vi "Create AIs.vi"(0 "reference in":refnum<class "Stand.lvclass">, 11 "error in (no error)":errorcluster) -> (4 "reference out":refnum<class "Stand.lvclass">, 15 "error out":errorcluster)   [LabVIEW 2019, in "Stand.lvclass"]
uses:
  Stand.lvclass
  C:/Users/ANENKOV_V1/Desktop/src/Proccess_class/Proccess.lvclass
  C:/Users/ANENKOV_V1/Desktop/src/Device_class/Device.lvclass
  Stand.lvclass/Stand.ctl
  TypeDef/CalibrationData.ctl
  TypeDef/GUI Setting Channel.ctl
  TypeDef/GUI AI Ranges.ctl
  TypeDef/Scale Data.ctl
  Device_class/Device.lvclass/Device.ctl
  Proccess_class/Proccess.lvclass/Proccess.ctl
  SV_Puplisher_class/SV_Publisher.lvclass/SV_Publisher.ctl
  AI_class/AI.lvclass
  Proccess_class/TAGs.ctl
  PiecedLinearScale_class/Scale_PiecedLinear.lvclass
  TypeDef/ConfigAnalogComp.ctl
  AI_class/AI Alarm Type.ctl
  PiecedLinearScale_class/Scale_PiecedLinear.lvclass/Scale_PiecedLinear.ctl
  AI_class/AI.lvclass/AI.ctl
  AnalogComparator_class/AnalogComparator.lvclass/AnalogComparator.ctl
  0edcd56b-ce9e-46cf-b3ab-c0e0e087750b.vi
  <vilib>/Utility/error.llb/Clear Errors.vi
  SV_Puplisher_class/Set SV.vi/1ae5d02c-efd0-450a-8aa4-8388e25d05bc.vi
  AnalogComparator_class/SetConfig.vi
  ConfigInterface_class/ConfigInterface.lvclass
  Proccess_class/Proccess.lvclass
  Device_class/Device.lvclass
  SV_Puplisher_class/SV_Publisher.lvclass
  AnalogComparator_class/AnalogComparator.lvclass
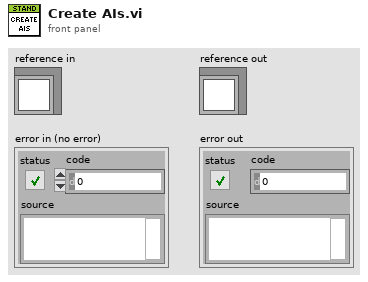
[diagram p1: front panel]
types:
  T1 = typedef "CalibrationData.ctl" = cluster{"Channels":T2[], "Scales":T4[]}
  T2 = typedef "GUI Setting Channel.ctl" = cluster{"Name":string, "AI Ranges":T3, "ScaleIndex":u32}
  T3 = typedef "GUI AI Ranges.ctl" = cluster{"HI":bool, "HIHI":bool, "LO":bool, "LOLO":bool, "HIHI VAL":dbl, "HI VAL":dbl, "LO VAL":dbl, "LOLO VAL":dbl, "MAX RAW":dbl, "MIN RAW":dbl, "MAX SCALED":dbl, "MIN SCALED":dbl}
  T4 = typedef "Scale Data.ctl" = cluster{"index":i32, "Name":string, "X":dbl[], "Y":dbl[]}
  T5 = typedef "Proccess.lvclass/TAGs.ctl" = cluster{"TAG":string, "PTAG":string, "DESC":string}
  T6 = typedef "ConfigAnalogComp.ctl" = cluster{"Threshold":dbl, "Hysteresis":dbl, "Invert":bool, "Enable":bool, "LockEn":bool}
  T7 = typedef "AnalogComparator.lvclass/AI Alarm Type.ctl" = enum16{"RAW MAX", "RAW MIN", "HIHI", "HI", "LO", "LOLO"}
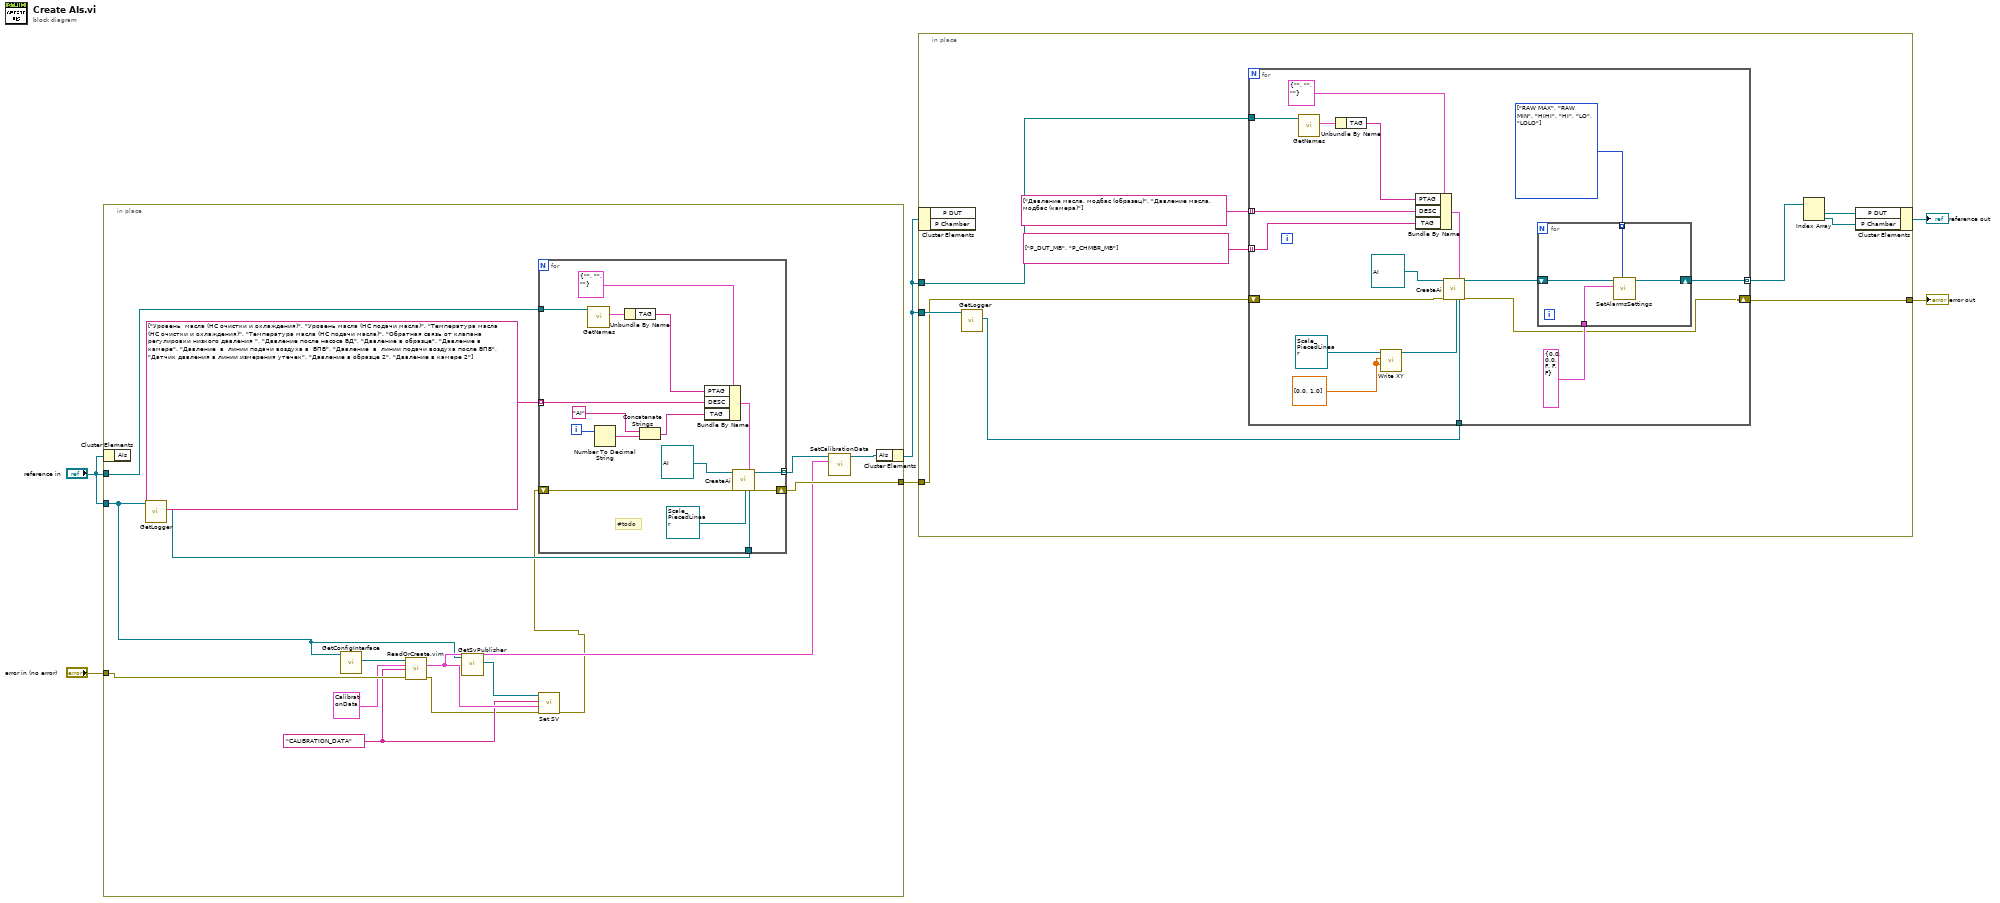
[diagram p0: block diagram]
diagram:
  n1 = in-place {
    in-place-border: "error in (no error)" -> [w15]
    in-place-border: "reference in" -> [w20]
    in-place-border: "reference in" -> [w16]
    in-place-border: [w18] -> w4
    w9 = "CALIBRATION_DATA" ("Name")
    n2 = in-place-cluster #1("reference in") -> ()  [unwired: 1 out]
    n3 = call "GetLogger.vi"("Proccess in"=w16) -> ("Logger"=w19:refnum<class "Logger.lvclass">)  [unwired: 10 in]
    n4 = call "GetConfigInterface.vi"("Device in"=w16) -> ("ConfigInterface"=w11:refnum<class "ConfigInterface.lvclass">)  [unwired: 10 in]
    n5 = call "ReadOrCreate.vim"("reference in"=w11, "Type and Defaults"=T1 {"Channels"=[{"Name"="AI0", "AI Ranges"={"HI"=FALSE, "HIHI"=FALSE, "LO"=FALSE, "LOLO"=FALSE, "HIHI VAL"=0.0, "HI VAL"=90.0, "LO VAL"=10.0, "LOLO VAL"=0.0, "MAX RAW"=20.0, "MIN RAW"=4.0, "MAX SCALED"=20.0, "MIN SCALED"=4.0}, "ScaleIndex"=0}, {"Name"="AI1", "AI Ranges"={"HI"=FALSE, "HIHI"=FALSE, "LO"=FALSE, "LOLO"=FALSE, "HIHI VAL"=0.0, "HI VAL"=90.0, "LO VAL"=10.0, "LOLO VAL"=0.0, "MAX RAW"=20.0, "MIN RAW"=4.0, "MAX SCALED"=20.0, "MIN SCALED"=4.0}, "ScaleIndex"=0}, {"Name"="AI2", "AI Ranges"={"HI"=FALSE, "HIHI"=FALSE, "LO"=FALSE, "LOLO"=FALSE, "HIHI VAL"=0.0, "HI VAL"=90.0, "LO VAL"=10.0, "LOLO VAL"=0.0, "MAX RAW"=20.0, "MIN RAW"=4.0, "MAX SCALED"=20.0, "MIN SCALED"=4.0}, "ScaleIndex"=0}, {"Name"="AI3", "AI Ranges"={"HI"=FALSE, "HIHI"=FALSE, "LO"=FALSE, "LOLO"=FALSE, "HIHI VAL"=0.0, "HI VAL"=90.0, "LO VAL"=10.0, "LOLO VAL"=0.0, "MAX RAW"=20.0, "MIN RAW"=4.0, "MAX SCALED"=20.0, "MIN SCALED"=4.0}, "ScaleIndex"=0}, {"Name"="AI4", "AI Ranges"={"HI"=FALSE, "HIHI"=FALSE, "LO"=FALSE, "LOLO"=FALSE, "HIHI VAL"=0.0, "HI VAL"=90.0, "LO VAL"=10.0, "LOLO VAL"=0.0, "MAX RAW"=20.0, "MIN RAW"=4.0, "MAX SCALED"=20.0, "MIN SCALED"=4.0}, "ScaleIndex"=0}, {"Name"="AI5", "AI Ranges"={"HI"=FALSE, "HIHI"=FALSE, "LO"=FALSE, "LOLO"=FALSE, "HIHI VAL"=0.0, "HI VAL"=90.0, "LO VAL"=10.0, "LOLO VAL"=0.0, "MAX RAW"=20.0, "MIN RAW"=4.0, "MAX SCALED"=20.0, "MIN SCALED"=4.0}, "ScaleIndex"=0}, {"Name"="AI6", "AI Ranges"={"HI"=FALSE, "HIHI"=FALSE, "LO"=FALSE, "LOLO"=FALSE, "HIHI VAL"=0.0, "HI VAL"=90.0, "LO VAL"=10.0, "LOLO VAL"=0.0, "MAX RAW"=20.0, "MIN RAW"=4.0, "MAX SCALED"=20.0, "MIN SCALED"=4.0}, "ScaleIndex"=0}, {"Name"="AI7", "AI Ranges"={"HI"=FALSE, "HIHI"=FALSE, "LO"=FALSE, "LOLO"=FALSE, "HIHI VAL"=0.0, "HI VAL"=90.0, "LO VAL"=10.0, "LOLO VAL"=0.0, "MAX RAW"=20.0, "MIN RAW"=4.0, "MAX SCALED"=20.0, "MIN SCALED"=4.0}, "ScaleIndex"=0}, {"Name"="AI8", "AI Ranges"={"HI"=FALSE, "HIHI"=FALSE, "LO"=FALSE, "LOLO"=FALSE, "HIHI VAL"=0.0, "HI VAL"=90.0, "LO VAL"=10.0, "LOLO VAL"=0.0, "MAX RAW"=20.0, "MIN RAW"=4.0, "MAX SCALED"=20.0, "MIN SCALED"=4.0}, "ScaleIndex"=0}, {"Name"="AI9", "AI Ranges"={"HI"=FALSE, "HIHI"=FALSE, "LO"=FALSE, "LOLO"=FALSE, "HIHI VAL"=0.0, "HI VAL"=90.0, "LO VAL"=10.0, "LOLO VAL"=0.0, "MAX RAW"=20.0, "MIN RAW"=4.0, "MAX SCALED"=20.0, "MIN SCALED"=4.0}, "ScaleIndex"=0}, {"Name"="AI10", "AI Ranges"={"HI"=FALSE, "HIHI"=FALSE, "LO"=FALSE, "LOLO"=FALSE, "HIHI VAL"=0.0, "HI VAL"=90.0, "LO VAL"=10.0, "LOLO VAL"=0.0, "MAX RAW"=20.0, "MIN RAW"=4.0, "MAX SCALED"=20.0, "MIN SCALED"=4.0}, "ScaleIndex"=0}], "Scales"=[]} ("CalibrationData"), "Name"=w9, "error in (no error)"=w15) -> ("Data"=w17:T1, "error out"=w7:errorcluster)  [unwired: 7 in, 3 out]
    n6 = call "GetSvPublisher.vi"("Device in"=w16) -> ("SV_Publisher.lvclass"=w10:refnum<class "SV_Publisher.lvclass">)  [unwired: 10 in]
    n7 = call "Set SV.vi"("error in (no error)"=w7, "SV Value"=w17, "SV Name"=w9, "SV_Publisher in"=w10) -> ("error out"=w12:errorcluster)  [unwired: 6 in, 1 out]
    n8 = for {
      tunnel: [w22] -> w14 mode=indexing
      shift-right: [w32] -> w18
      shift-left: w12 -> [w33]
      tunnel: string[] ["Уровень  масла (НС очистки и охлаждения)", "Уровень масла (НС подачи масла)", "Температура масла (НС очистки и охлаждения)", "Температура масла (НС подачи масла)", "Обратная связь от клапана регулировки низкого давления ", "Давление после насоса ВД", "Давление в образце", "Давление в камере", "Давление  в  линии подачи воздуха в  БПВ", "Давление  в  линии подачи воздуха после БПВ", "Датчик давления в линии измерения утечек", "Давление в образце 2", "Давление в камере 2"] ("ParentName") -> [w28] mode=indexing
      tunnel: w20 -> [w25]
      tunnel: w19 -> [w24]
      i -> [w37]
      # "#todo"
      n9 = call "GetNames.vi"("Proccess in"=w25) -> ("Tags"=w27:T5)  [unwired: 10 in]
      n10 = Number To Decimal String(number=w37) -> (decimal integer string=w36:string)  [unwired: 1 in]
      n11 = Unbundle By Name(w27) -> ("TAG"=w26:string)
      n12 = Concatenate Strings("AI" ("string"), w36) -> (w29:string)
      n13 = Bundle By Name(cluster=T5 {"TAG"="", "PTAG"="", "DESC"=""} ("Tags"), "PTAG"=w26, "DESC"=w28, "TAG"=w29) -> (w30:T5)
      n14 = call "CreateAi.vi"("AI in"=refnum<class "AI.lvclass"> refnum ("Sig_AI"), "error in (no error)"=w33, "Scale"=refnum<class "Scale_PiecedLinear.lvclass"> refnum, "Tags"=w30, "Logger"=w24) -> ("AI out"=w22:refnum<class "AI.lvclass">, "error out"=w32:errorcluster)  [unwired: 13 in]
    }
    n15 = call "SetCalibrationData.vi"("AIs in"=w14, "data"=w17) -> ("AIs out"=w13:refnum<class "AI.lvclass">[])  [unwired: 13 in]
    n16 = in-place-cluster #1("AIs"=w13) -> (w3:refnum<class "Stand.lvclass">)
  }
  n17 = in-place {
    in-place-border: w4 -> [w42]
    in-place-border: w3 -> [w46]
    in-place-border: w3 -> [w43]
    in-place-border: [w44] -> w2
    n18 = in-place-cluster #2(w3) -> ()  [unwired: 2 out]
    n19 = call "GetLogger.vi"("Proccess in"=w43) -> ("Logger"=w45:refnum<class "Logger.lvclass">)  [unwired: 10 in]
    n20 = for {
      tunnel: [w49] -> w41 mode=indexing
      shift-right: [w48] -> w44
      shift-left: w42 -> [w64]
      tunnel: string[] ["Давление масла, модбас (образец)", "Давление масла, модбас (камера)"] ("ParentName") -> [w61] mode=indexing
      tunnel: w46 -> [w58]
      tunnel: w45 -> [w57]
      tunnel: string[] ["P_DUT_MB", "P_CHMBR_MB"] ("ParentName") -> [w53] mode=indexing
      w52 = T7[] [enum."RAW MAX", enum."RAW MIN", enum."HIHI", enum."HI", enum."LO", enum."LOLO"] items=["RAW MAX", "RAW MIN", "HIHI", "HI", "LO", "LOLO"] ("Array")
      w56 = dbl[] [0.0, 1.0] ("Y")
      n21 = call "GetNames.vi"("Proccess in"=w58) -> ("Tags"=w60:T5)  [unwired: 10 in]
      n22 = Unbundle By Name(w60) -> ("TAG"=w59:string)
      n23 = call "Write XY.vi"("X"=w56, "Y"=w56, "Scale_PiecedLinear in"=refnum<class "Scale_PiecedLinear.lvclass"> refnum) -> ("Scale_PiecedLinear out"=w54:refnum<class "Scale_PiecedLinear.lvclass">)  [unwired: 8 in]
      n24 = Bundle By Name(cluster=T5 {"TAG"="", "PTAG"="", "DESC"=""} ("Tags"), "PTAG"=w59, "DESC"=w61, "TAG"=w53) -> (w62:T5)
      n25 = call "CreateAi.vi"("AI in"=refnum<class "AI.lvclass"> refnum ("Sig_AI"), "error in (no error)"=w64, "Scale"=w54, "Tags"=w62, "Logger"=w57) -> ("AI out"=w50:refnum<class "AI.lvclass">, "error out"=w48:errorcluster)  [unwired: 13 in]
      n26 = for {
        tunnel: w52 -> [w69] mode=indexing
        tunnel: T6 {"Threshold"=0.0, "Hysteresis"=0.0, "Invert"=FALSE, "Enable"=FALSE, "LockEn"=FALSE} ("SettinganalogComp") -> [w68]
        shift-right: [w66] -> w49
        shift-left: w50 -> [w67]
        n27 = call "SetAlarmsSettings.vi"("TYPE"=w69, "SettinganalogComp"=w68, "Sig_AI in"=w67) -> ("Sig_AI out"=w66:refnum<class "AI.lvclass">)  [unwired: 8 in]
      }
    }
    n28 = Index Array(array=w41) -> (element #1=w40:refnum<class "AI.lvclass">, element #2=w39:refnum<class "AI.lvclass">)  [unwired: 2 in]
    n29 = in-place-cluster #2("P DUT"=w40, "P Chamber"=w39) -> (→"reference out":refnum<class "Stand.lvclass">)
  }
  "error out" <- w2
